vi "Signal Set Data.vi"(8 "error in (no error)":errorcluster, 10 "Data":refnum<data-value>, 11 "Signal DVR in":refnum<data-value>) -> (0 "error out":errorcluster, 3 "Signal DVR out":refnum<data-value>)   [LabVIEW 2010, in "MDSplus.lvlib"]
uses:
  <vilib>/MDSplus/Library/MDSplus.lvlib
  <vilib>/MDSplus/Classes/Data_Class/Data.lvclass
  <vilib>/MDSplus/Classes/Data_Class/Compound_Class/Signal_Class/Signal.lvclass
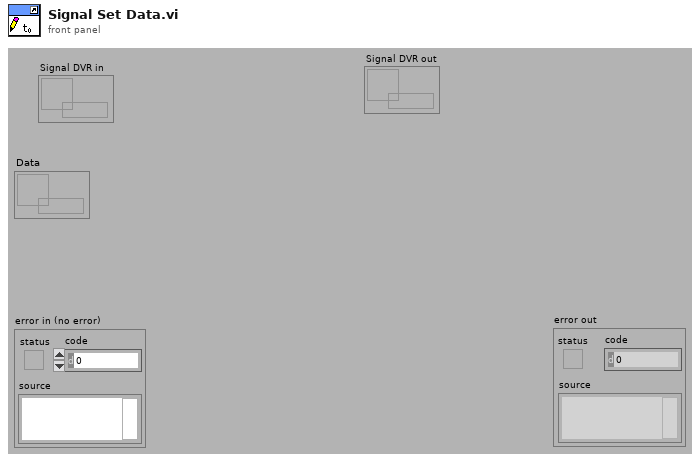
[diagram p1: front panel]
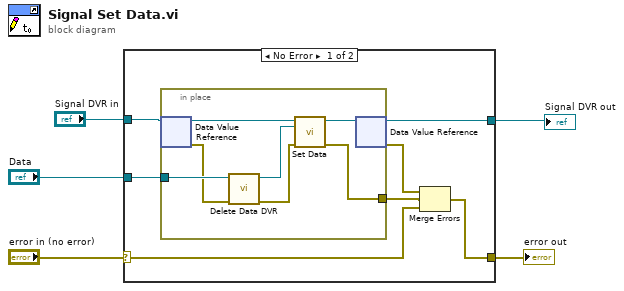
[diagram p0: block diagram]
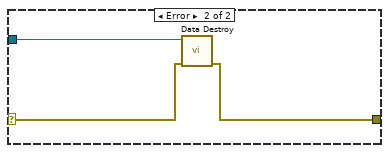
[diagram p2: hidden frame]
diagram:
  n1 = case shown="No Error" "error in (no error)" {
    selector: "error in (no error)" -> [w12 w21]
    tunnel: [w10 w20] -> w5
    tunnel: "Data" -> [w9 w22]
    tunnel: "Signal DVR in" -> [w8 _]
    tunnel: [w7 _] -> w1
    frame No Error {
      n2 = in-place {
        in-place-border: w9 -> [w19]
        in-place-border: [w13] -> w6
        n3 = in-place-dvr #1(w8) -> (w17:refnum<class "Signal.lvclass">, w18:errorcluster)
        n4 = call <vilib>:"Delete Data DVR.vi"("error in (no error)"=w18, "Data DVR in"=w19) -> ("error out"=w14:errorcluster, "Data out"=w15:refnum<class "Data.lvclass">)  [unwired: 8 in]
        n5 = call <vilib>:"Set Data.vi"("error in (no error)"=w14, "Data"=w15, "Signal in"=w17) -> ("error out"=w13:errorcluster, "Signal out"=w16:refnum<class "Signal.lvclass">)  [unwired: 7 in]
        n6 = in-place-dvr #1(w16) -> (w7:refnum<data-value>, w11:errorcluster)
      }
      n7 = Merge Errors(w11, w6, w12) -> (w10:errorcluster)
    }
    frame Error {
      n8 = call <vilib>:"Data Destroy.vi"("error in (no error)"=w21, "Data DVR in"=w22) -> ("error out"=w20:errorcluster)  [unwired: 9 in]
    }
  }
  "error out" <- w5
  "Signal DVR out" <- w1
